vi "Read_Instr.vi"(8 "error in (no error)":errorcluster caption="entrée d'erreur (pas d'erreur)", 11 "Class Instrument Power_Supply en entrée":refnum<class "Class Instrument Power_Supply.lvclass">) -> (0 "error out":errorcluster caption="sortie d'erreur", 3 "Class Instrument Power_Supply en sortie":refnum<class "Class Instrument Power_Supply.lvclass">)   [LabVIEW 2020, in "Library Instrument & Equipement.lvlib" / "Library Instruments.lvlib" / "Class Instrument Power_Supply.lvclass"]
uses:
  Class Instrument Power_Supply.lvclass
  Class Instrument Power_Supply.lvclass/Class Instrument Power_Supply.ctl
  Instrument (Default)/Class Instrument (Default).lvclass
  Power_Supply/Power_Supply (Default)/Power_Supply (Default).lvclass
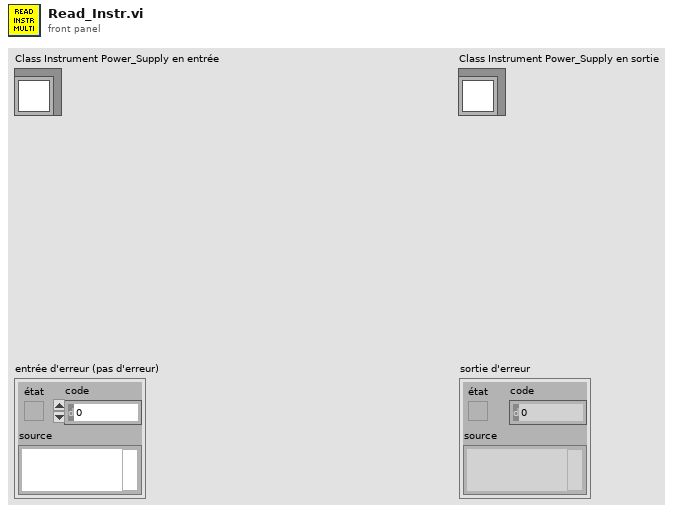
[diagram p1: front panel]
types:
  T1 = cluster{"Power":dbl, "Voltage":dbl, "Current":dbl}
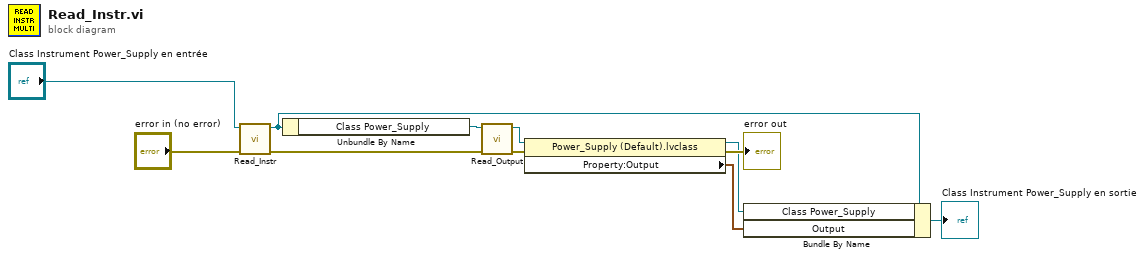
[diagram p0: block diagram]
diagram:
  n1 = call-parent "Read_Instr.vi"("error in (no error)"="error in (no error)", "Class Instrument (Default) en entrée"="Class Instrument Power_Supply en entrée") -> ("error out"=w9:errorcluster, "Class Instrument (Default) en sortie"=w2:refnum<class "Class Instrument Power_Supply.lvclass">)  [unwired: 8 in]
  n2 = Unbundle By Name(w2) -> ("Class Power_Supply"=w8:refnum<class "Power_Supply (Default).lvclass">)
  n3 = call-dynamic "Read_Output.vi"("error in (no error)"=w9, "Power_Supply (Default) en entrée"=w8) -> ("error out"=w6:errorcluster, "Power_Supply (Default) en sortie"=w4:refnum<class "Power_Supply (Default).lvclass">)  [unwired: 8 in]
  n4 = property class="Power_Supply (Default).lvclass"(reference=w4, error in=w6) -> (reference out=w1:refnum<class "Power_Supply (Default).lvclass">, error out=→"error out":errorcluster, "Property:Output"=w7:T1)
  n5 = Bundle By Name(cluster=w2, "Class Power_Supply"=w1, "Output"=w7) -> (→"Class Instrument Power_Supply en sortie":refnum<class "Class Instrument Power_Supply.lvclass">)
